vi "StateMachine.vi"() -> ()   [LabVIEW 2014]
uses:
  StateMachineControl.ctl
panel:
  in  "stop":bool
  out "motor on time [ms]":u32
  out "millisecond timer":u32
  out "motor on":bool
  in  "motor timer  [ms]":u32
  in  "user button":bool
  in  "index pulse":bool
  out "state":T1
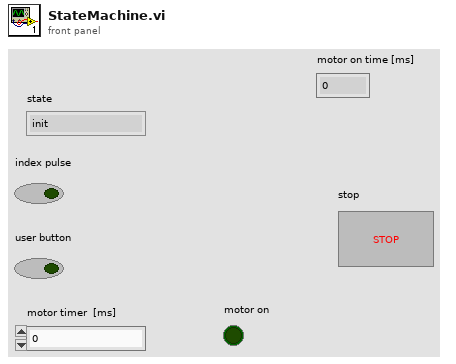
[diagram p1: front panel]
types:
  T1 = typedef "StateMachineControl.ctl" = enum16{"init", "waiting for pulse", "waiting for button", "running motor", "shutdown"}
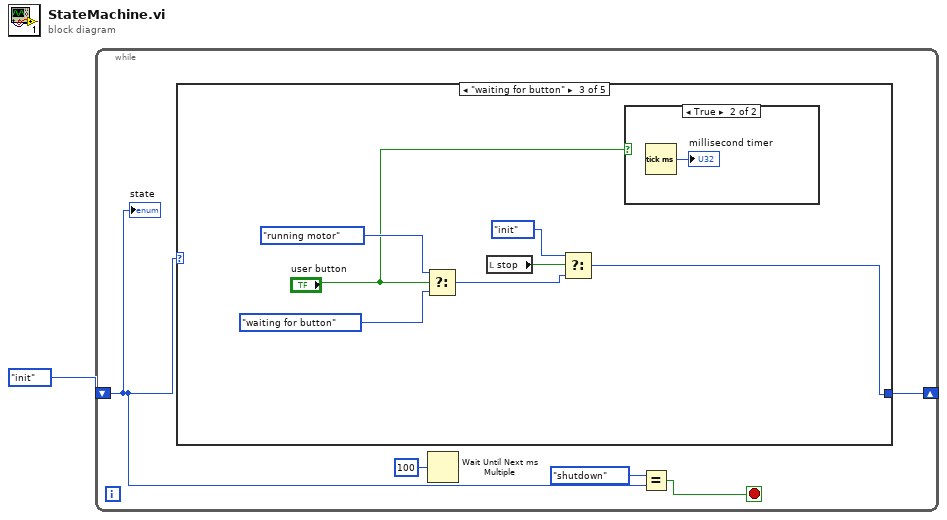
[diagram p0: block diagram]
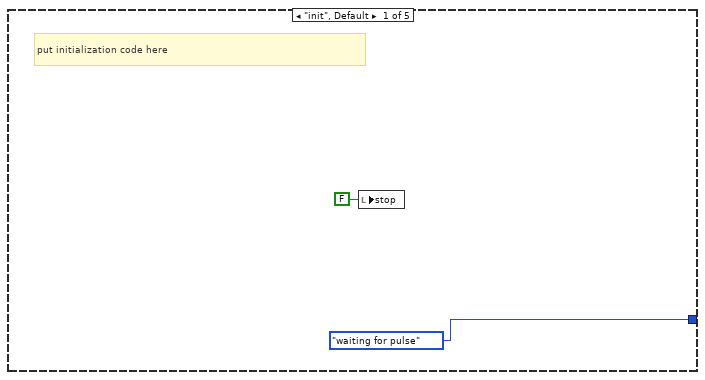
[diagram p2: hidden frame]
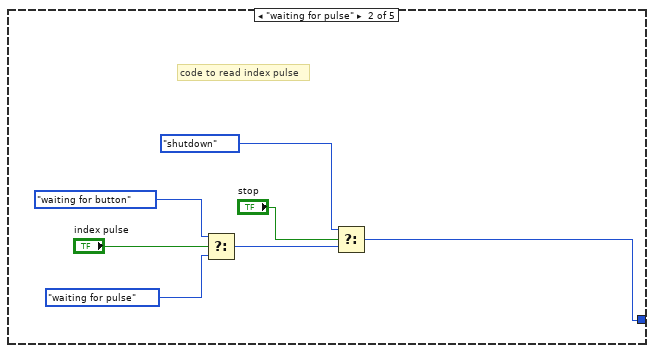
[diagram p3: hidden frame]
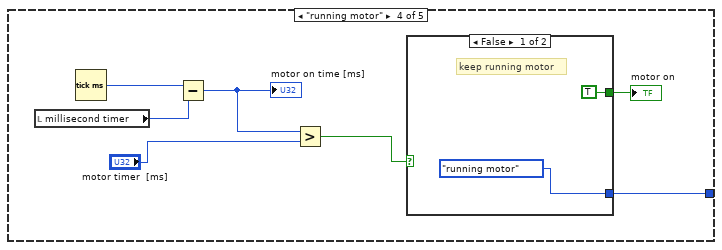
[diagram p5: hidden frame]
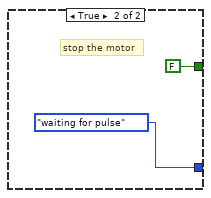
[diagram p6: hidden frame]
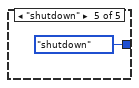
[diagram p7: hidden frame]
diagram:
  n1 = while {
    shift-right: [w6] -> _
    shift-left: StateMachineControl."init" ("state") -> [w2]
    stop <- w4 stop-if-true
    n2 = case shown="\"waiting for button\"" w2 {
      tunnel: [StateMachineControl."waiting for pulse" ("state") w9 w16 w24 StateMachineControl."shutdown" ("state")] -> w6
      frame "init", Default {
        # "put initialization code here"
        n3 = local write "stop"(FALSE ("stop")) -> ()
      }
      frame "waiting for pulse" {
        # "code to read index pulse"
        n4 = Select(t=StateMachineControl."waiting for button" ("x"), s="index pulse", f=StateMachineControl."waiting for pulse" ("x")) -> (s? t:f=w12:T1)
        n5 = Select(t=StateMachineControl."shutdown" ("state"), s="stop", f=w12) -> (s? t:f=w9:T1)
      }
      frame "waiting for button" {
        n6 = Select(t=StateMachineControl."running motor" ("x"), s="user button", f=StateMachineControl."waiting for button" ("x")) -> (s? t:f=w17:T1)
        n7 = local read "stop"() -> (w19:bool)
        n8 = Select(t=StateMachineControl."init" ("state"), s=w19, f=w17) -> (s? t:f=w16:T1)
        n9 = case shown="True" "user button" {
          frame False {
          }
          frame True {
            n10 = Tick Count (ms)() -> (millisecond timer value=→"millisecond timer":u32)
          }
        }
      }
      frame "running motor" {
        n11 = local read "millisecond timer"() -> (w30:u32)
        n12 = Tick Count (ms)() -> (millisecond timer value=w29:u32)
        n13 = Subtract(x=w29, y=w30) -> (x-y=w27:u32)
        "motor on time [ms]" <- w27
        n14 = Greater?(x=w27, y="motor timer  [ms]") -> (0:w26:bool)
        n15 = case shown="False" w26 {
          tunnel: [TRUE ("motor on") FALSE ("motor on")] -> w25
          tunnel: [StateMachineControl."running motor" ("state") StateMachineControl."waiting for pulse" ("state")] -> w24
          frame False {
            # "keep running motor"
          }
          frame True {
            # "stop the motor"
          }
        }
        "motor on" <- w25
      }
      frame "shutdown" {
      }
    }
    n16 = Wait Until Next ms Multiple(millisecond multiple=u32 100) -> ()  [unwired: 1 out]
    n17 = Equal?(x=StateMachineControl."shutdown", y=w2) -> (x = y?=w4:bool)
    "state" <- w2
  }
